vi "Read.vi"(7 "I2C Channel":u8, 8 "Error In":errorcluster, 10 "I2C Slave Address (0)":u8 format="%x", 11 "LINX Resource":T2) -> (0 "Error Out":errorcluster, 2 "Acceleration Data (g)":T1, 3 "LINX Resource":T2)   [LabVIEW 2020, in "LMH-LINX.lvlib" / "MMA8451.lvlib"]
doc: "Read X, Y and Z axis of acceleration data (in g's) from the MMA8451."
uses:
  MMA8451.lvlib
  Private/Type Defs/LINX Ref.ctl
  Private/Type Defs/Platform.ctl
  Private/Type Defs/Interface.ctl
  Private/Device/Type Defs/LINX Device Config.ctl
  Private/Device/Type Defs/TCP Config.ctl
  Private/Device/Type Defs/Channels.ctl
  Private/Type Defs/Peripherals/I2C/EOF.ctl
  Private/Local IO/LinxI2cWrite.vi
  Utilities/Check Channel.vi
  Private/Utilties/Generate Error.vi
  LMH-LINX.lvlib
  Private/Device/Device.lvlib
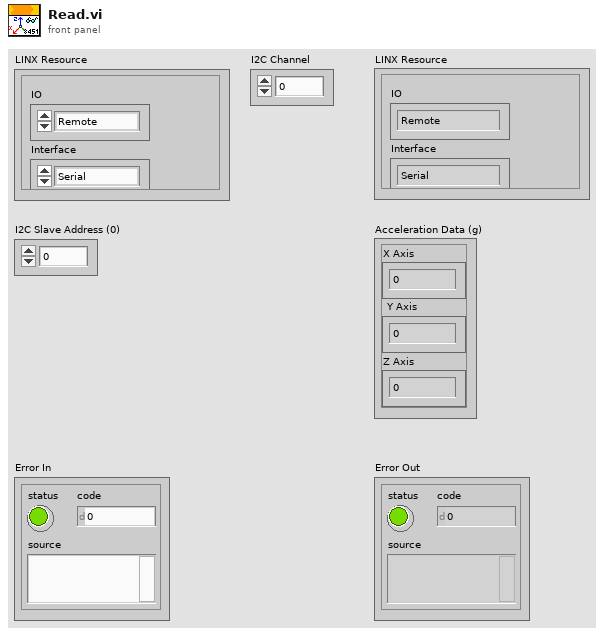
[diagram p1: front panel]
types:
  T1 = cluster{"X Axis":dbl, "Y Axis":dbl, "Z Axis":dbl}
  T2 = typedef "LMH-LINX.lvlib/LINX Ref.ctl" = cluster{"IO":T3, "Interface":T4, "LINX Device Config":T5}
  T3 = typedef "LMH-LINX.lvlib/Platform.ctl" = enum16{"Remote", "Local"}
  T4 = typedef "LMH-LINX.lvlib/Interface.ctl" = enum16{"Serial", "TCP"}
  T5 = typedef "Device.lvlib/LINX Device Config.ctl" = cluster{"Interface":T4, "COM Port":refnum<visa-resource-name>, "TCP Configuration":T6, "Device Family":u8, "Device ID":u8, "Device Name":string, "TCP Ref":refnum<k5>, "Channels":T7}
  T6 = typedef "Device.lvlib/TCP Config.ctl" = cluster{"IP Address":string, "Port":u16}
  T7 = typedef "LMH-LINX.lvlib/Channels.ctl" = cluster{"DI":u8[], "DO":u8[], "AI":u8[], "AO":u8[], "PWM":u8[], "QE":u8[], "UART":u8[], "I2C 2":u8[], "SPI":u8[], "CAN":u8[], "Servo":u8[], "AI Ref (V)":dbl, "AI Resolution (Bits)":u8, "AO Ref (V)":dbl, "AO Resolution (Bits)":u8}
  T8 = typedef "LMH-LINX.lvlib/EOF.ctl" = enum8{"Stop", "Restart", "Restart No Stop", "No Stop"}
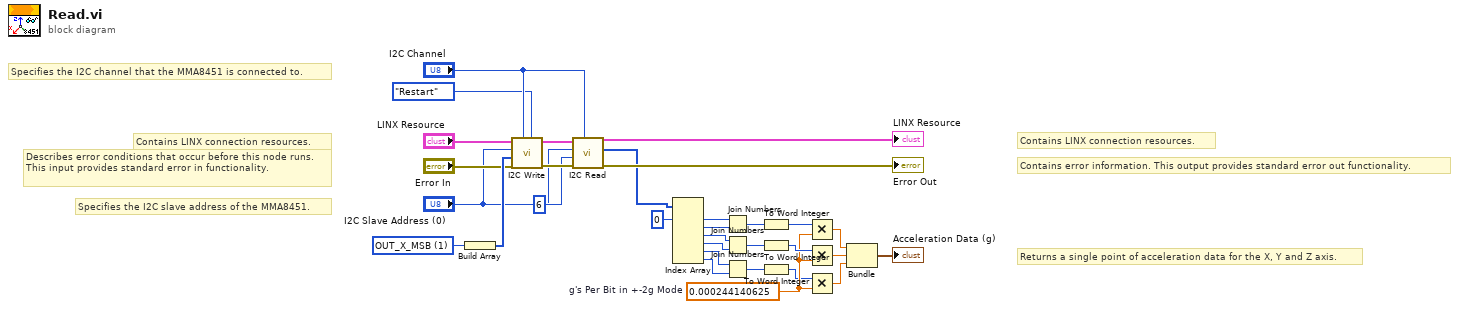
[diagram p0: block diagram]
diagram:
  w21 = u8 1 items=["OUT_X_MSB"=1, "SYSMOD"=11, "WHOAMI"=13, "XYZ_DATA_CFG"=14, "PL_STATUS"=16, "PL_CFG"=17, "CTRL_REG1"=42, "CTRL_REG2"=43, "CTRL_REG4"=45, "CTRL_REG5"=46] ("MMA8451 REG_OUT_X_MSB")
  w6 = 0.000244140625  # g's Per Bit in +-2g Mode
  # "Specifies the I2C slave address of the MMA8451."
  # "Specifies the I2C channel that the MMA8451 is connected to."
  # "Returns a single point of acceleration data for the X, Y and Z axis."
  # "Contains LINX connection resources."
  # "Contains error information. This output provides standard error out functionality."
  # "Contains LINX connection resources."
  # "Describes error conditions that occur before this node runs. This input provides standard error in functionality."
  n1 = Build Array(w21) -> (w28:u8[])
  n2 = call "I2C Write.vi"("EOF"=EOF."Restart", "I2C Channel"="I2C Channel", "Error In"="Error In", "Data"=w28, "I2C Slave Address (0)"="I2C Slave Address (0)", "LINX Resource"="LINX Resource") -> ("Error Out"=w30:errorcluster, "LINX Resource"=w31:T2)  [unwired: 4 in]
  n3 = call "I2C Read.vi"("I2C Channel"="I2C Channel", "Error In"=w30, "Bytes To Read"=u8 6, "I2C Slave Address (0)"="I2C Slave Address (0)", "LINX Resource"=w31) -> ("Error Out"=→"Error Out":errorcluster, "Data"=w18:u8[], "LINX Resource"=→"LINX Resource":T2)  [unwired: 4 in]
  n4 = Index Array(array=w18, index #1=0 ("index")) -> (element #1=w19:u8, element #2=w13:u8, element #3=w12:u8, element #4=w11:u8, element #5=w10:u8, element #6=w9:u8)  [unwired: 5 in]
  n5 = Join Numbers(hi=w19, lo=w13) -> ((hi.lo)=w17:u16)
  n6 = Join Numbers(hi=w12, lo=w11) -> ((hi.lo)=w16:u16)
  n7 = Join Numbers(hi=w10, lo=w9) -> ((hi.lo)=w15:u16)
  n8 = To Word Integer(number=w17) -> (16bit integer=w8:i16)
  n9 = To Word Integer(number=w16) -> (16bit integer=w7:i16)
  n10 = To Word Integer(number=w15) -> (16bit integer=w5:i16)
  n11 = Multiply(x=w8, y=w6) -> (x*y=w4:dbl)
  n12 = Multiply(x=w7, y=w6) -> (x*y=w3:dbl)
  n13 = Multiply(x=w5, y=w6) -> (x*y=w2:dbl)
  n14 = Bundle(w4, w3, w2) -> (→"Acceleration Data (g)":cluster{dbl, dbl, dbl})  [unwired: 1 in]
